vi "Set Single Control.vi"(8 "error in (no error)":errorcluster, 9 "New Value":variant, 10 "Indicator Name":string, 11 "Controls_Mgr in":refnum<class "Controls_Mgr.lvclass">) -> (0 "error out":errorcluster, 3 "Controls_Mgr out":refnum<class "Controls_Mgr.lvclass">)   [LabVIEW 2015, in "Generic Module Library.lvlib" / "Template G_Module.lvlib" / "Controls_Mgr.lvclass"]
uses:
  Controls_Mgr.lvclass
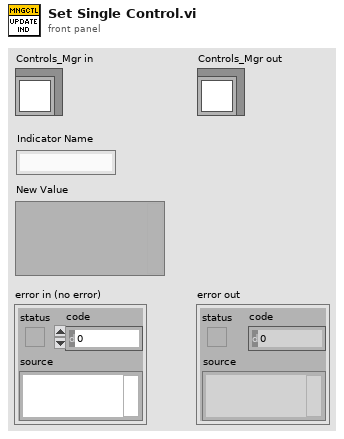
[diagram p1: front panel]
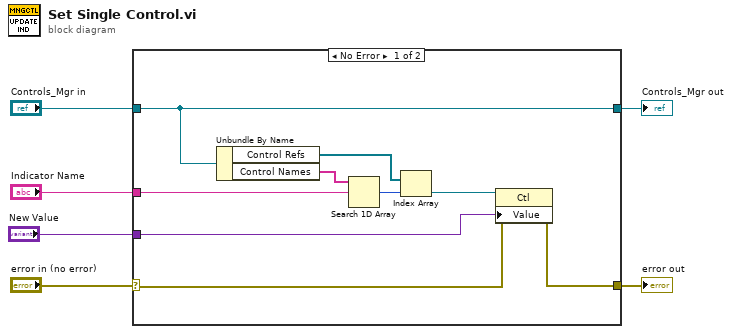
[diagram p0: block diagram]
diagram:
  n1 = case shown="No Error" "error in (no error)" {
    selector: "error in (no error)" -> [w8 w17]
    tunnel: [w7 w17] -> w5
    tunnel: [w11 w16] -> w3
    tunnel: "Controls_Mgr in" -> [w11 w16]
    tunnel: "New Value" -> [w9 _]
    tunnel: "Indicator Name" -> [w10 _]
    frame No Error {
      n2 = Unbundle By Name(w11) -> ("Control Refs"=w13:refnum<vi>[], "Control Names"=w15:string[])
      n3 = Search 1D Array(1D array=w15, element=w10) -> (index of element=w14:i32)  [unwired: 1 in]
      n4 = Index Array(array=w13, index=w14) -> (element=w12:refnum<vi>)
      n5 = property class="Ctl"(reference=w12, error in=w8, "Value"=w9) -> (error out=w7:errorcluster)  [unwired: 1 out]
    }
    frame Error {
    }
  }
  "error out" <- w5
  "Controls_Mgr out" <- w3
